vi "SingleMoleFinder.vi"(0 "Color Plane (IntensityExtraction)":i32(ring)=6 items=["Red", "Green", "Blue", "Hue", "Saturation", "Luminance", "Value", "Intensity"], 1 "Kernel (SmothingGaussian)":sgl[][](array[numeric])=[[1.0, 2.0, 4.0, 2.0, 1.0], [2.0, 4.0, 8.0, 4.0, 2.0], [4.0, 8.0, 16.0, 8.0, 4.0], [2.0, 4.0, 8.0, 4.0, 2.0], [1.0, 2.0, 4.0, 2.0, 1.0]], 2 "Divider (SmothingGaussian)":sgl, 3 "Kernel (Convolution)":sgl[][](array[numeric])=[[-1.0, -1.0, -1.0, -1.0, -1.0], [-1.0, -1.0, -1.0, -1.0, -1.0], [-1.0, -1.0, 30.0, -1.0, -1.0], [-1.0, -1.0, -1.0, -1.0, -1.0], [-1.0, -1.0, -1.0, -1.0, -1.0]], 4 "Divider (Convolution)":sgl, 5 "Method (AutoTresholdMomentClustering)":i32(ring)=3 items=["clustering", "entropy", "metric", "moments", "inter-class variance"], 6 "Look For (AutoTresholdMomentClustering)":u32(ring) items=["Bright Objects", "Dark Objects"], 7 "error in":errorcluster, 8 "Operator (LogarithmicSmoother)":T3(ring)=enum."Log", 9 "X Value (LogarithmicSmoother)":sgl=1.5, 10 "Operation (closeObjects)":T2(ring)=enum."PClose", 11 "Structuring Element (closeObjects)":i32[][](array[numeric])=[[0, 1, 1, 1, 0], [1, 1, 1, 1, 1], [1, 1, 1, 1, 1], [1, 1, 1, 1, 1], [0, 1, 1, 1, 0]], 12 "Square/Hexa (Square) (closeObjects)":bool, 13 "Connectivity 4/8 (8) (RemoveBorderObjects)":bool=TRUE, 14 "Square/Hexa (Square) (RemoveSmallObjects)":bool=TRUE, 15 "Connectivity 4/8 (8) (RemoveSmallObjects)":bool=TRUE, 16 "Low Pass/High Pass (Low) (RemoveSmallObjects)":bool, 17 "Connectivity 4/8 (8) (FillHoles)":bool=TRUE, 18 "Min Radius (CircleDetection)":sgl=15.0, 19 "Max Radius (CircleDetection)":sgl=50.0, 21 "Keep/Remove Particles (Particle Filter 1)":bool=TRUE, 22 "Connectivity 4/8 (8) (Particle Filter 1)":bool=TRUE, 23 "Selection Values (Particle Filter 1)":T1(array[cluster])=[{"Measurement Parameter"=1, "Range Lower Value"=0.0, "Range Upper Value"=0.0, "Range"=FALSE, "Measurement Type"=FALSE}, {"Measurement Parameter"=0, "Range Lower Value"=15.0, "Range Upper Value"=100.0, "Range"=FALSE, "Measurement Type"=FALSE}] {"Measurement Parameter" items=["Center of Mass X", "Center of Mass Y", "First Pixel X", "First Pixel Y", "Bounding Rect Left", "Bounding Rect Top", "Bounding Rect Right", "Bounding Rect Bottom", "Max Feret Diameter Start X", "Max Feret Diameter Start Y", "Max Feret Diameter End X", "Max Feret Diameter End Y", "Max Horiz. Segment Length Left", "Max Horiz. Segment Length Right", "Max Horiz. Segment Length Row", "-", "Bounding Rect Width", "Bounding Rect Height", "Bounding Rect Diagonal", "Perimeter", "Convex Hull Perimeter", "Holes' Perimeter", "Max Feret Diameter", "Equivalent Ellipse Major Axis", "Equivalent Ellipse Minor Axis", "Equivalent Ellipse Minor Axis (Feret)", "Equivalent Rect Long Side", "Equivalent Rect Short Side", "Equivalent Rect Diagonal", "Equivalent Rect Short Side (Feret)", "Average Horiz. Segment Length", "Average Vert. Segment Length", "Hydraulic Radius", "Waddel Disk Diameter", "-", "Area", "Holes' Area", "Particle & Holes' Area", "Convex Hull Area", "Image Area", "-", "Number of Holes", "Number of Horiz. Segments", "Number of Vert. Segments", "-", "Orientation", "Max Feret Diameter Orientation", "-", "% Area/Image Area", "% Area/(Particle & Holes' Area)", "Ratio of Equivalent Ellipse Axes", "Ratio of Equivalent Rect Sides", "-", "Elongation Factor", "Compactness Factor", "Heywood Circularity Factor", "Type Factor", "-", "Sum X", "Sum Y", "Sum XX", "Sum XY", "Sum YY", "Sum XXX", "Sum XXY", "Sum XYY", "Sum YYY", "-", "Moment of Inertia XX", "Moment of Inertia XY", "Moment of Inertia YY", "Moment of Inertia XXX", "Moment of Inertia XXY", "Moment of Inertia XYY", "Moment of Inertia YYY", "Norm. Moment of Inertia XX", "Norm. Moment of Inertia XY", "Norm. Moment of Inertia YY", "Norm. Moment of Inertia XXX", "Norm. Moment of Inertia XXY", "Norm. Moment of Inertia XYY", "Norm. Moment of Inertia YYY", "Hu Moment 1", "Hu Moment 2", "Hu Moment 3", "Hu Moment 4", "Hu Moment 5", "Hu Moment 6", "Hu Moment 7"]}, 24 "Connectivity 4/8 (8) (ParticleTable)":bool=TRUE, 25 "Pixel Measurements (ParticleTable)":i32[](array[ring])=[0, 1, 2, 3, 4, 5, 6, 7, 8, 9, 10, 11, 12, 13, 14, 16, 17, 18, 19, 20, 21, 22, 23, 24, 25, 26, 27, 28, 29, 30, 31, 32, 33, 35, 36, 37, 38, 39, 41, 42, 43, 45, 46, 48, 49, 50, 51, 53, 54, 55, 56, 58, 59, 60, 61, 62, 63, 64, 65, 66, 68, 69, 70, 71, 72, 73, 74, 75, 76, 77, 78, 79, 80, 81, 82, 83, 84, 85, 86, 87, 88] items=["Center of Mass X", "Center of Mass Y", "First Pixel X", "First Pixel Y", "Bounding Rect Left", "Bounding Rect Top", "Bounding Rect Right", "Bounding Rect Bottom", "Max Feret Diameter Start X", "Max Feret Diameter Start Y", "Max Feret Diameter End X", "Max Feret Diameter End Y", "Max Horiz. Segment Length Left", "Max Horiz. Segment Length Right", "Max Horiz. Segment Length Row", "-", "Bounding Rect Width", "Bounding Rect Height", "Bounding Rect Diagonal", "Perimeter", "Convex Hull Perimeter", "Holes' Perimeter", "Max Feret Diameter", "Equivalent Ellipse Major Axis", "Equivalent Ellipse Minor Axis", "Equivalent Ellipse Minor Axis (Feret)", "Equivalent Rect Long Side", "Equivalent Rect Short Side", "Equivalent Rect Diagonal", "Equivalent Rect Short Side (Feret)", "Average Horiz. Segment Length", "Average Vert. Segment Length", "Hydraulic Radius", "Waddel Disk Diameter", "-", "Area", "Holes' Area", "Particle & Holes' Area", "Convex Hull Area", "Image Area", "-", "Number of Holes", "Number of Horiz. Segments", "Number of Vert. Segments", "-", "Orientation", "Max Feret Diameter Orientation", "-", "% Area/Image Area", "% Area/(Particle & Holes' Area)", "Ratio of Equivalent Ellipse Axes", "Ratio of Equivalent Rect Sides", "-", "Elongation Factor", "Compactness Factor", "Heywood Circularity Factor", "Type Factor", "-", "Sum X", "Sum Y", "Sum XX", "Sum XY", "Sum YY", "Sum XXX", "Sum XXY", "Sum XYY", "Sum YYY", "-", "Moment of Inertia XX", "Moment of Inertia XY", "Moment of Inertia YY", "Moment of Inertia XXX", "Moment of Inertia XXY", "Moment of Inertia XYY", "Moment of Inertia YYY", "Norm. Moment of Inertia XX", "Norm. Moment of Inertia XY", "Norm. Moment of Inertia YY", "Norm. Moment of Inertia XXX", "Norm. Moment of Inertia XXY", "Norm. Moment of Inertia XYY", "Norm. Moment of Inertia YYY", "Hu Moment 1", "Hu Moment 2", "Hu Moment 3", "Hu Moment 4", "Hu Moment 5", "Hu Moment 6", "Hu Moment 7"]) -> (20 "Nb Circles (CircleDetection)":i32, 26 "Circles Data (CircleDetection)":T5(array[cluster]), 27 "error out":errorcluster)   [LabVIEW 2010]
uses:
  <vilib>/vision/NI_Vision_Development_Module.lvlib
panel:
  out "Image Out":T4(plugin-control)
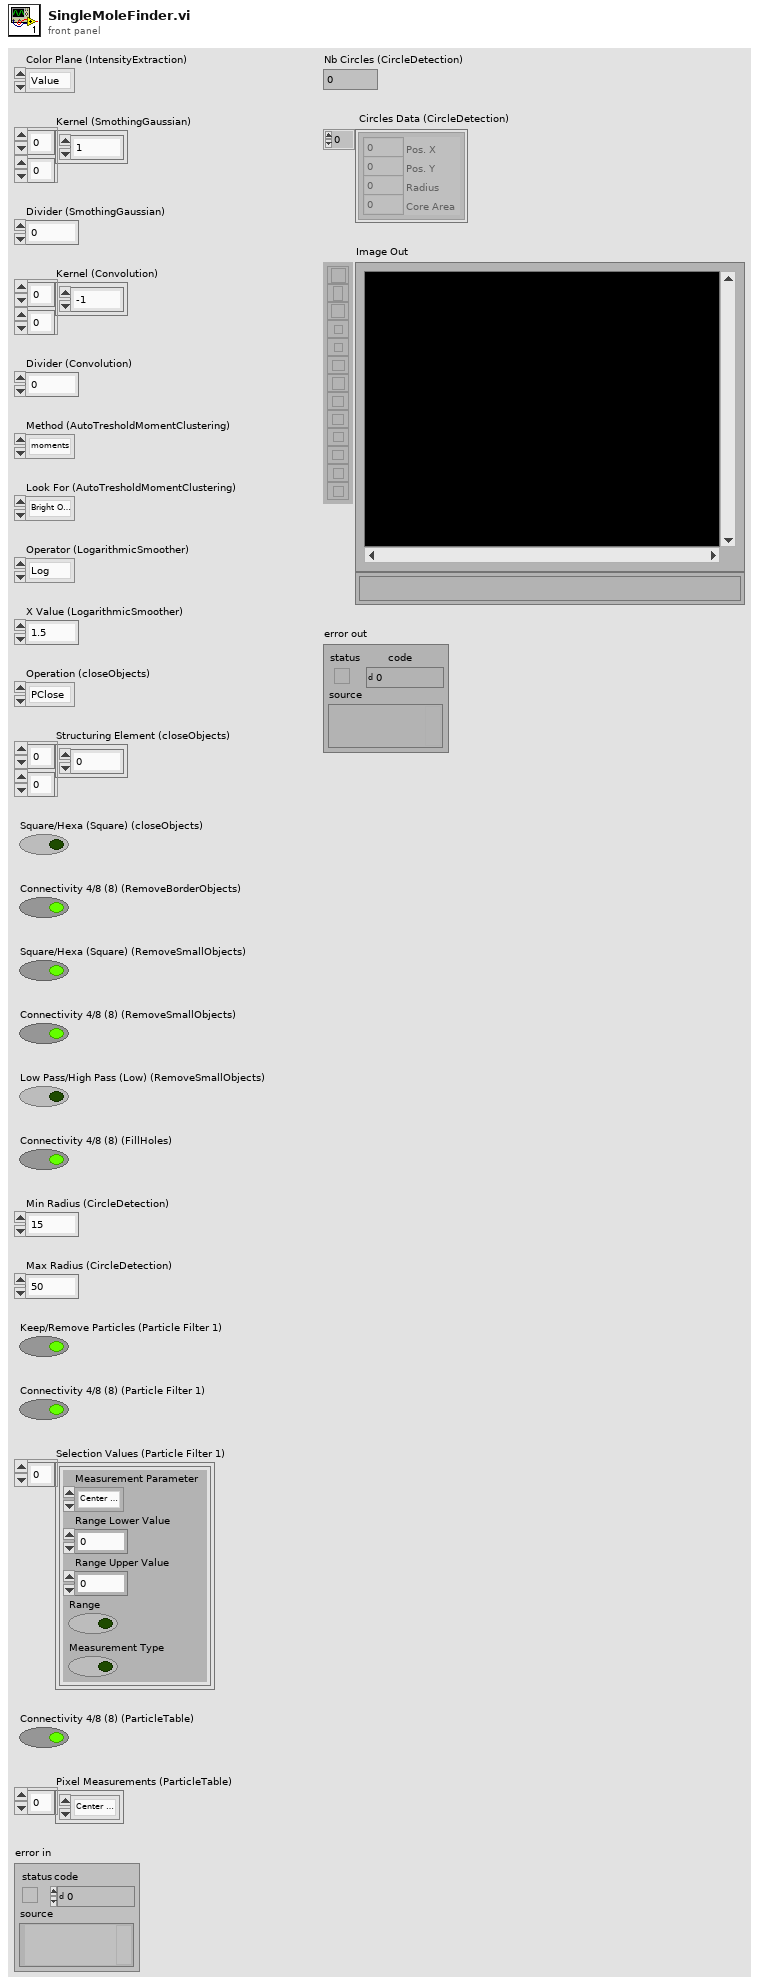
[diagram p1: front panel]
types:
  T1 = cluster{"Measurement Parameter":i32, "Range Lower Value":dbl, "Range Upper Value":dbl, "Range":bool, "Measurement Type":bool}[]
  T2 = enum32{"AutoM", "Close", "Dilate", "Erode", "Gradient", "Gradient out", "Gradient in", "Hit miss", "Open", "PClose", "POpen", "Thick", "Thin"}
  T3 = enum32{"Linear", "Log", "Exp", "Square", "Square root", "Power X", "Power 1/X"}
  T4 = typedef "IMAQ Image.ctl" = refnum<image>
  T5 = cluster{"Pos. X":i32, "Pos. Y":i32, "Radius":i32, "Core Area":i32}[]
  T6 = typedef "Image Type" = u32
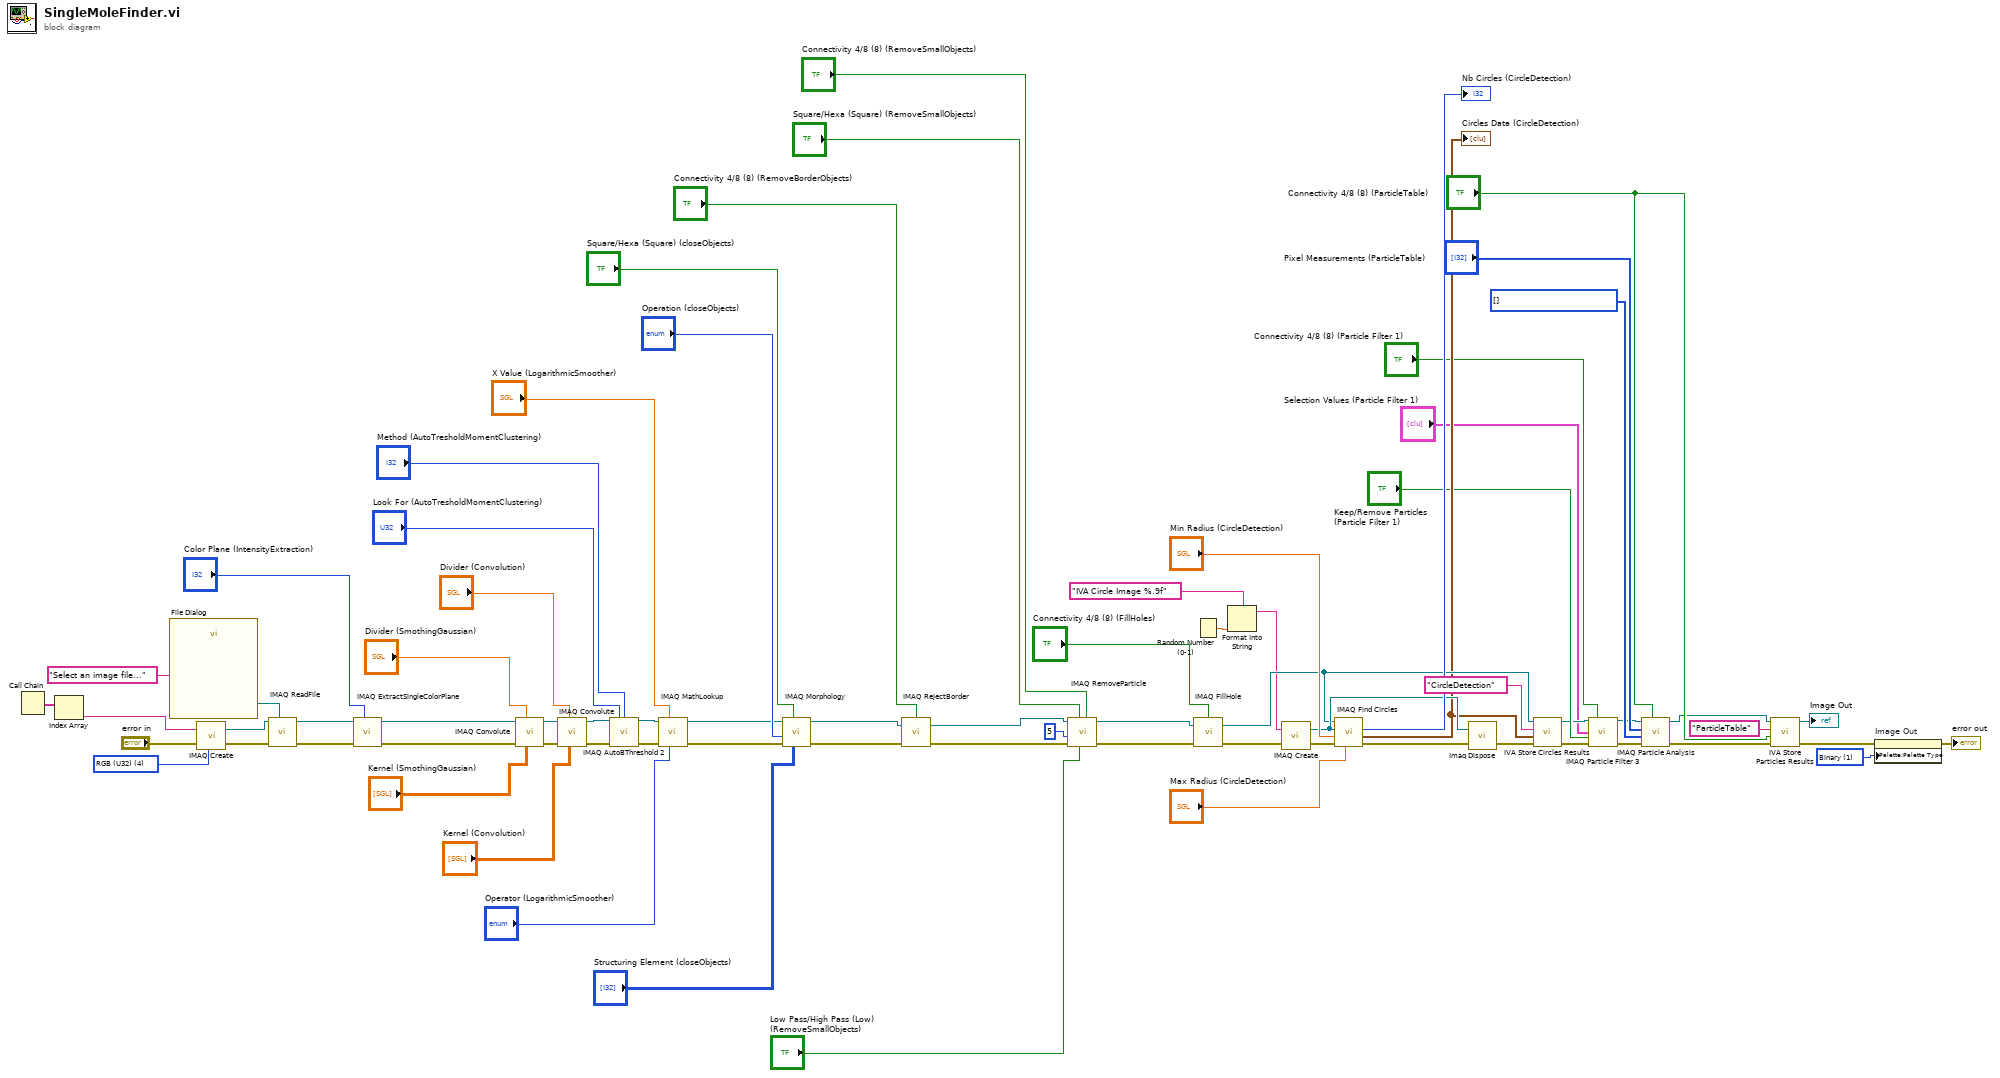
[diagram p0: block diagram]
diagram:
  w3 = u32 1 items=["Grayscale", "Binary", "Gradient", "Rainbow", "Temperature", "User Defined"] ("Palette")
  w11 = i32[] [] items=["Center of Mass X", "Center of Mass Y", "First Pixel X", "First Pixel Y", "Bounding Rect Left", "Bounding Rect Top", "Bounding Rect Right", "Bounding Rect Bottom", "Max Feret Diameter Start X", "Max Feret Diameter Start Y", "Max Feret Diameter End X", "Max Feret Diameter End Y", "Max Horiz. Segment Length Left", "Max Horiz. Segment Length Right", "Max Horiz. Segment Length Row", "-", "Bounding Rect Width", "Bounding Rect Height", "Bounding Rect Diagonal", "Perimeter", "Convex Hull Perimeter", "Holes' Perimeter", "Max Feret Diameter", "Equivalent Ellipse Major Axis", "Equivalent Ellipse Minor Axis", "Equivalent Ellipse Minor Axis (Feret)", "Equivalent Rect Long Side", "Equivalent Rect Short Side", "Equivalent Rect Diagonal", "Equivalent Rect Short Side (Feret)", "Average Horiz. Segment Length", "Average Vert. Segment Length", "Hydraulic Radius", "Waddel Disk Diameter", "-", "Area", "Holes' Area", "Particle & Holes' Area", "Convex Hull Area", "Image Area", "-", "Number of Holes", "Number of Horiz. Segments", "Number of Vert. Segments", "-", "Orientation", "Max Feret Diameter Orientation", "-", "% Area/Image Area", "% Area/(Particle & Holes' Area)", "Ratio of Equivalent Ellipse Axes", "Ratio of Equivalent Rect Sides", "-", "Elongation Factor", "Compactness Factor", "Heywood Circularity Factor", "Type Factor", "-", "Sum X", "Sum Y", "Sum XX", "Sum XY", "Sum YY", "Sum XXX", "Sum XXY", "Sum XYY", "Sum YYY", "-", "Moment of Inertia XX", "Moment of Inertia XY", "Moment of Inertia YY", "Moment of Inertia XXX", "Moment of Inertia XXY", "Moment of Inertia XYY", "Moment of Inertia YYY", "Norm. Moment of Inertia XX", "Norm. Moment of Inertia XY", "Norm. Moment of Inertia YY", "Norm. Moment of Inertia XXX", "Norm. Moment of Inertia XXY", "Norm. Moment of Inertia XYY", "Norm. Moment of Inertia YYY", "Hu Moment 1", "Hu Moment 2", "Hu Moment 3", "Hu Moment 4", "Hu Moment 5", "Hu Moment 6", "Hu Moment 7"] ("Real-World Measurements")
  w68 = T6 4 items=["Grayscale (U8)", "Grayscale (I16)", "Grayscale (SGL)", "Complex (CSG)", "RGB (U32)", "HSL (U32)", "RGB (U64)", "Grayscale (U16)"] ("Image Type")
  n1 = Call Chain() -> (call chain=w72:string[])
  n2 = Index Array(array=w72) -> (element=w71:string)  [unwired: 1 in]
  n3 = call "File Dialog"("prompt"="Select an image file...") -> ("selected path"=w69:path)  [unwired: 6 in, 8 out]
  n4 = call "IMAQ Create"("Image Name"=w71, "Image Type"=w68, "error in (no error)"="error in") -> ("New Image"=w75:T4, "error out"=w74:errorcluster)  [unwired: 1 in, 1 out]
  n5 = call "IMAQ ReadFile"("File Path"=w69, "error in (no error)"=w74, "Image"=w75) -> ("error out"=w65:errorcluster, "Image Out"=w66:T4)  [unwired: 2 in, 5 out]
  n6 = call "IMAQ ExtractSingleColorPlane"("Color Plane"="Color Plane (IntensityExtraction)", "error in (no error)"=w65, "Image Src"=w66) -> ("error out"=w62:errorcluster, "Image Dst Out"=w63:T4)  [unwired: 1 in, 6 out]
  n7 = call "IMAQ Convolute"("Kernel"="Kernel (SmothingGaussian)", "Divider (kernel sum)"="Divider (SmothingGaussian)", "error in (no error)"=w62, "Image Src"=w63) -> ("error out"=w58:errorcluster, "Image Dst Out"=w59:T4)  [unwired: 3 in, 3 out]
  n8 = call "IMAQ Convolute"("Kernel"="Kernel (Convolution)", "Divider (kernel sum)"="Divider (Convolution)", "error in (no error)"=w58, "Image Src"=w59) -> ("error out"=w56:errorcluster, "Image Dst Out"=w55:T4)  [unwired: 3 in, 3 out]
  n9 = call "IMAQ AutoBThreshold 2"("Image Src"=w55, "Look For (Bright Objects)"="Look For (AutoTresholdMomentClustering)", "Method (clustering)"="Method (AutoTresholdMomentClustering)", "error in (no error)"=w56) -> ("Image Dst Out"=w50:T4, "error out"=w49:errorcluster)  [unwired: 4 in, 6 out]
  n10 = call "IMAQ MathLookup"("Operator"="Operator (LogarithmicSmoother)", "X Value"="X Value (LogarithmicSmoother)", "error in (no error)"=w49, "Image Src"=w50) -> ("error out"=w44:errorcluster, "Image Dst Out"=w45:T4)  [unwired: 3 in, 3 out]
  n11 = call "IMAQ Morphology"("Structuring Element"="Structuring Element (closeObjects)", "Square/Hexa (Square)"="Square/Hexa (Square) (closeObjects)", "error in (no error)"=w44, "Operation"="Operation (closeObjects)", "Image Src"=w45) -> ("error out"=w41:errorcluster, "Image Dst Out"=w42:T4)  [unwired: 2 in, 3 out]
  n12 = call "IMAQ RejectBorder"("error in (no error)"=w41, "Image Src"=w42, "Connectivity 4/8 (8)"="Connectivity 4/8 (8) (RemoveBorderObjects)") -> ("error out"=w35:errorcluster, "Image Dst Out"=w36:T4)  [unwired: 1 in, 2 out]
  n13 = call "IMAQ RemoveParticle"("Connectivity 4/8 (8)"="Connectivity 4/8 (8) (RemoveSmallObjects)", "Low Pass/High Pass (Low)"="Low Pass/High Pass (Low) (RemoveSmallObjects)", "Square/Hexa (Square)"="Square/Hexa (Square) (RemoveSmallObjects)", "error in (no error)"=w35, "Number of Erosion"=5, "Image Src"=w36) -> ("error out"=w32:errorcluster, "Image Dst Out"=w33:T4)  [unwired: 1 in, 3 out]
  n14 = Random Number (0-1)() -> (number: 0 to 1=w18:dbl)
  n15 = call "IMAQ FillHole"("error in (no error)"=w32, "Image Src"=w33, "Connectivity 4/8 (8)"="Connectivity 4/8 (8) (FillHoles)") -> ("error out"=w26:errorcluster, "Image Dst Out"=w23:T4)  [unwired: 1 in, 2 out]
  n16 = Format Into String(format string="IVA Circle Image %.9f" ("Image Name"), w18) -> (resulting string=w20:string)  [unwired: 2 in, 1 out]
  n17 = call "IMAQ Create"("Image Name"=w20, "error in (no error)"=w26) -> ("New Image"=w28:T4, "error out"=w27:errorcluster)  [unwired: 2 in, 1 out]
  n18 = call "IMAQ Find Circles"("Max Radius"="Max Radius (CircleDetection)", "error in (no error)"=w27, "Min Radius"="Min Radius (CircleDetection)", "Image Dst"=w28, "Image Src"=w23) -> ("error out"=w25:errorcluster, "Circles Data"=w21:T5, "Nb Circles"=→"Nb Circles (CircleDetection)":i32)  [unwired: 4 out]
  "Circles Data (CircleDetection)" <- w21
  n19 = call "Imaq Dispose"("Image"=w28, "error in (no error)"=w25) -> ("error out"=w24:errorcluster)  [unwired: 1 in, 3 out]
  n20 = call <vilib>:"IVA Store Circles Results.vi"("error in (no error)"=w24, "Circles Data"=w21, "Step Name"="CircleDetection", "Image in"=w23) -> ("error out"=w14:errorcluster, "Image dup"=w15:T4)  [unwired: 6 out]
  n21 = call "IMAQ Particle Filter 3"("Image Src"=w15, "Connectivity 4/8 (8)"="Connectivity 4/8 (8) (Particle Filter 1)", "Selection Values"="Selection Values (Particle Filter 1)", "Keep/Remove Particles (F)"="Keep/Remove Particles (Particle Filter 1)", "error in (no error)"=w14) -> ("Image Dst Out"=w9:T4, "error out"=w10:errorcluster)  [unwired: 4 in, 5 out]
  n22 = call "IMAQ Particle Analysis"("Connectivity 4/8 (8)"="Connectivity 4/8 (8) (ParticleTable)", "error in (no error)"=w10, "Real-World Measurements"=w11, "Pixel Measurements"="Pixel Measurements (ParticleTable)", "Image"=w9) -> ("error out"=w5:errorcluster, "Image Out (duplicate)"=w7:T4)  [unwired: 5 out]
  n23 = call <vilib>:"IVA Store Particles Results.vi"("error in (no error)"=w5, "Connectivity 4/8 (8)"="Connectivity 4/8 (8) (ParticleTable)", "Step Name"="ParticleTable", "Image in"=w7) -> ("error out"=w2:errorcluster, "Image dup"=→"Image Out":T4)  [unwired: 6 out]
  n24 = property on="Image Out" class="ImageControl"(error in=w2, "Palette:Palette Type"=w3) -> (error out=→"error out":errorcluster)  [unwired: 1 in, 1 out]
